vi "Script Error.vi"(0 "Error?":bool, 1 "Reset Log":bool, 2 "Error Details":string, 3 "Error Code":i32, 4 "Line Number":i32) -> (5 "Error?":bool)   [LabVIEW 2014]
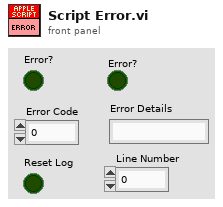
[diagram p1: front panel]
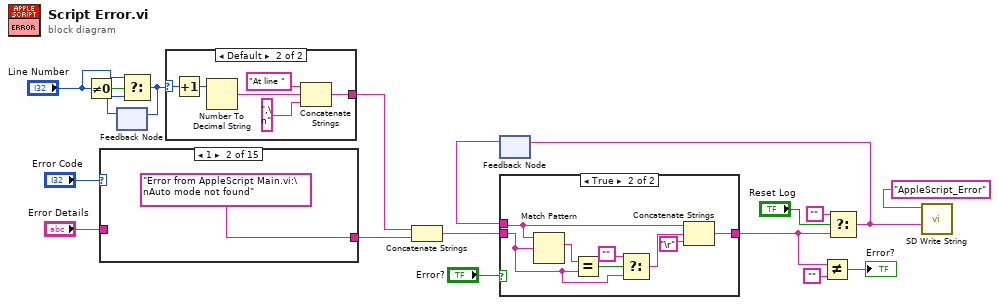
[diagram p0: block diagram]
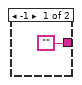
[diagram p2: hidden frame]
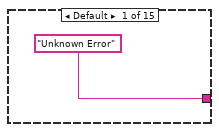
[diagram p4: hidden frame]
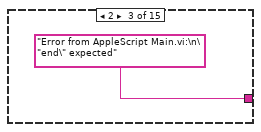
[diagram p5: hidden frame]
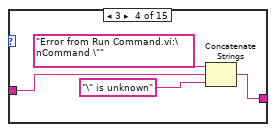
[diagram p6: hidden frame]
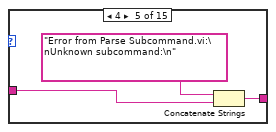
[diagram p7: hidden frame]
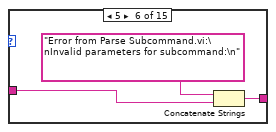
[diagram p8: hidden frame]
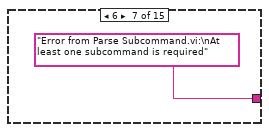
[diagram p9: hidden frame]
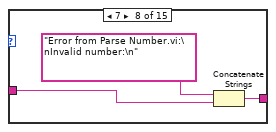
[diagram p10: hidden frame]
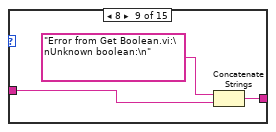
[diagram p11: hidden frame]
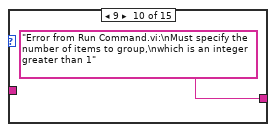
[diagram p12: hidden frame]
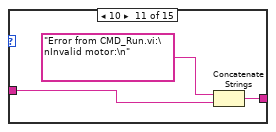
[diagram p13: hidden frame]
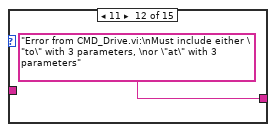
[diagram p14: hidden frame]
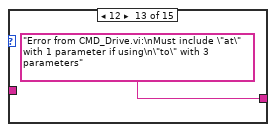
[diagram p15: hidden frame]
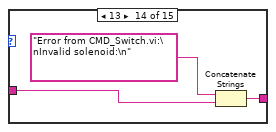
[diagram p16: hidden frame]
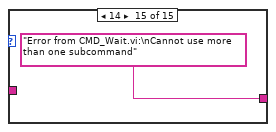
[diagram p17: hidden frame]
diagram:
  n1 = Not Equal To 0?(x="Line Number") -> (x != 0?=w7:bool)
  n2 = case shown="1" "Error Code" {
    tunnel: ["Unknown Error" "Error from AppleScript Main.vi:\nAuto mode not found" "Error from AppleScript Main.vi:\n\"end\" expected" w23 w26 w29 "Error from Parse Subcommand.vi:\nAt least one subcommand is required" w33 w36 "Error from Run Command.vi:\nMust specify the number of items to group,\nwhich is an integer greater than 1" w40 "Error from CMD_Drive.vi:\nMust include either \"to\" with 3 parameters, \nor \"at\" with 3 parameters" "Error from CMD_Drive.vi:\nMust include \"at\" with 1 parameter if using\n\"to\" with 3 parameters" w45 "Error from CMD_Wait.vi:\nCannot use more than one subcommand"] -> w12
    tunnel: "Error Details" -> [_ _ _ w24 w27 w30 _ w34 w37 _ w41 _ _ w46 _]
    frame Default {
    }
    frame 1 {
    }
    frame 2 {
    }
    frame 3 {
      n3 = Concatenate Strings("Error from Run Command.vi:\nCommand \"", w24, "\" is unknown" ("string")) -> (w23:string)
    }
    frame 4 {
      n4 = Concatenate Strings("Error from Parse Subcommand.vi:\nUnknown subcommand:\n", w27) -> (w26:string)
    }
    frame 5 {
      n5 = Concatenate Strings("Error from Parse Subcommand.vi:\nInvalid parameters for subcommand:\n", w30) -> (w29:string)
    }
    frame 6 {
    }
    frame 7 {
      n6 = Concatenate Strings("Error from Parse Number.vi:\nInvalid number:\n", w34) -> (w33:string)
    }
    frame 8 {
      n7 = Concatenate Strings("Error from Get Boolean.vi:\nUnknown boolean:\n", w37) -> (w36:string)
    }
    frame 9 {
    }
    frame 10 {
      n8 = Concatenate Strings("Error from CMD_Run.vi:\nInvalid motor:\n", w41) -> (w40:string)
    }
    frame 11 {
    }
    frame 12 {
    }
    frame 13 {
      n9 = Concatenate Strings("Error from CMD_Switch.vi:\nInvalid solenoid:\n", w46) -> (w45:string)
    }
    frame 14 {
    }
  }
  n10 = feedback #1() -> (w6:i32)  [unwired: 1 in]
  n11 = Select(t="Line Number", s=w7, f=w6) -> (s? t:f=w5:i32)
  n12 = feedback-in #1(w5) -> ()
  n13 = case shown="Default" w5 {
    selector: w5 -> [_ w51]
    tunnel: ["" w53] -> w11
    frame -1 {
    }
    frame Default {
      n14 = Increment(x=w51) -> (x+1=w50:i32)
      n15 = Number To Decimal String(number=w50) -> (decimal integer string=w55:string)  [unwired: 1 in]
      n16 = Concatenate Strings("At line " ("string"), w55, ",\n" ("string")) -> (w53:string)
    }
  }
  n17 = Concatenate Strings(w11, w12) -> (w9:string)
  n18 = feedback #2() -> (w10:string)  [unwired: 1 in]
  n19 = case shown="True" "Error?" {
    tunnel: w9 -> [_ w60]
    tunnel: w10 -> [w56 w62]
    tunnel: [w56 w64] -> w3
    frame False {
    }
    frame True {
      n20 = Match Pattern(string=w62, regular expression=w60) -> (match substring=w63:string)  [unwired: 1 in, 3 out]
      n21 = Equal?(x=w63, y=w60) -> (x = y?=w61:bool)
      n22 = Select(t="", s=w61, f=w60) -> (s? t:f=w58:string)
      n23 = Concatenate Strings(w62, w58, "\r") -> (w64:string)
    }
  }
  n24 = Not Equal?(x=w3, y="") -> (x != y?=→"Error?":bool)
  n25 = Select(t="", s="Reset Log", f=w3) -> (s? t:f=w16:string)
  n26 = feedback-in #2(w16) -> ()
  n27 = call <vilib>:"SD Write String.vi"("String"=w16, "Name"="AppleScript_Error") -> ()  [unwired: 8 in, 2 out]
